vi "Ex6_IteratingThroughArrayWithForloop.vi"() -> ()   [LabVIEW 2024]
panel:
  out "Array 2":dbl[](array[numeric])
  in  "Array":dbl[](array[numeric])
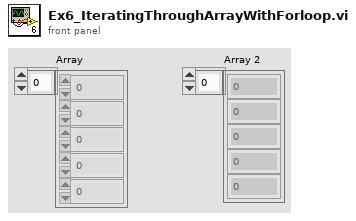
[diagram p1: front panel]
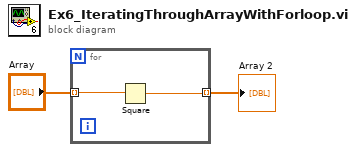
[diagram p0: block diagram]
diagram:
  n1 = for {
    tunnel: "Array" -> [w4] mode=indexing
    tunnel: [w3] -> w1 mode=indexing
    n2 = Square(x=w4) -> (x^2=w3:dbl)
  }
  "Array 2" <- w1
